vi "encapsulacion_Envio.vi"(4 "PORT":i32, 6 "prepend array or string size? (T)":bool, 7 "Numeric 2":u32, 9 "byte order (0:big-endian, network order)":T1(ring), 10 "Array":u8[](array[numeric]), 11 "UDP Network Connection in":refnum<k16>) -> (0 "error out":errorcluster)   [LabVIEW 2024]
panel:
  out "data string":string
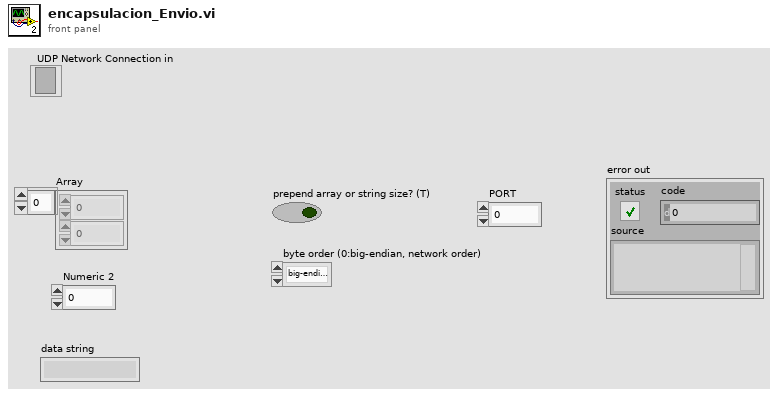
[diagram p1: front panel]
types:
  T1 = enum16{"big-endian, network order", "native, host order", "little-endian"}
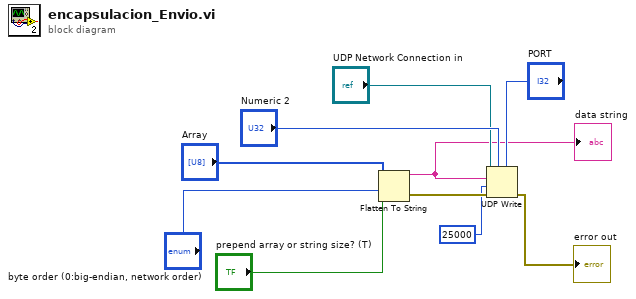
[diagram p0: block diagram]
diagram:
  n1 = Flatten To String(anything="Array", prepend array or string size? (T)="prepend array or string size? (T)", byte order (0:big-endian, network order)="byte order (0:big-endian, network order)") -> (data string=w1:string, error out=w7:errorcluster)  [unwired: 1 in, 1 out]
  "data string" <- w1
  n2 = UDP Write(address="Numeric 2", port or service name="PORT", connection ID="UDP Network Connection in", data in=w1, 8:w7, 9:25000) -> (error out=→"error out":errorcluster)  [unwired: 1 out]
